vi "TimeInterpVariant_GetNewestSample.vi"(11 "TimeInterpVariant":T1) -> (1 "IsPresent":bool, 2 "TimeStamp":dbl, 3 "OutputVariant":variant)   [LabVIEW 2019, in "Trajectory_Library.lvlib"]
doc: "Get the newest sample\n\nInputs:\n - TimeInterpVariant -- Input data cluster\n\nOutputs\n - OutputVariant -- Newest Variant. \n - TimeStamp -- Time for this sample (seconds)\n - IsPresent -- Returns TRUE if the buffer contains any data"
uses:
  TypeDef/TIME_INTERPOLATABLE_VARIANT.ctl
  Trajectory_Library.lvlib
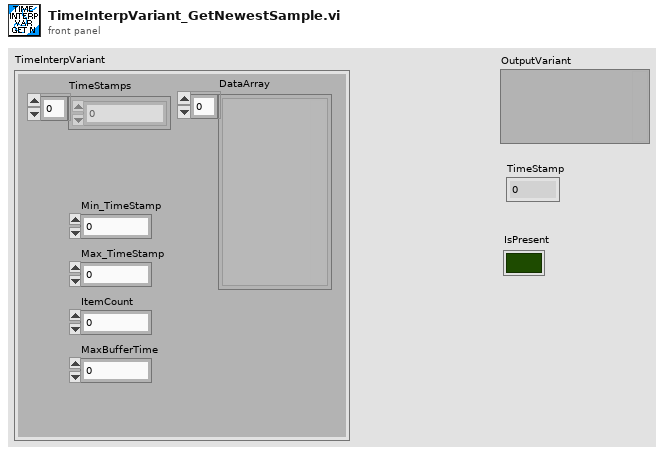
[diagram p1: front panel]
types:
  T1 = typedef "Trajectory_Library.lvlib/TIME_INTERPOLATABLE_VARIANT.ctl" = cluster{"TimeStamps":dbl[], "DataArray":variant[], "Min_TimeStamp":dbl, "Max_TimeStamp":dbl, "ItemCount":i32, "MaxBufferTime":dbl}
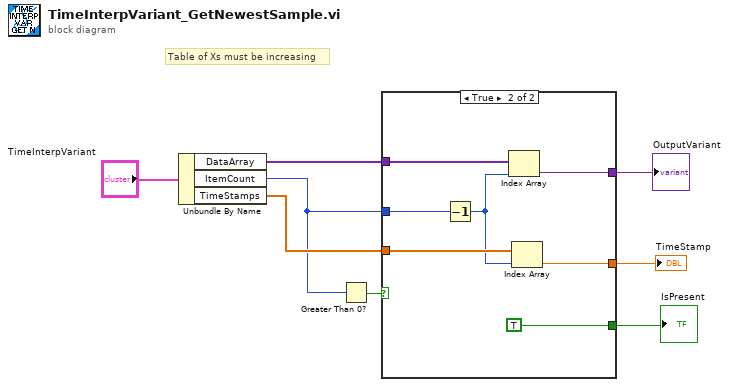
[diagram p0: block diagram]
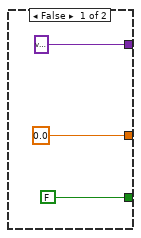
[diagram p2: hidden frame]
diagram:
  # "Table of Xs must be increasing"
  n1 = Unbundle By Name("TimeInterpVariant") -> ("DataArray"=w6:variant[], "ItemCount"=w4:i32, "TimeStamps"=w7:dbl[])
  n2 = Greater Than 0?(x=w4) -> (x > 0?=w5:bool)
  n3 = case shown="True" w5 {
    tunnel: [variant w15] -> w2
    tunnel: w4 -> [_ w13]
    tunnel: w7 -> [_ w17]
    tunnel: w6 -> [_ w18]
    tunnel: [FALSE TRUE] -> w3
    tunnel: [0.0 w16] -> w1
    frame False {
    }
    frame True {
      n4 = Decrement(x=w13) -> (x-1=w12:i32)
      n5 = Index Array(array=w18, index=w12) -> (element=w15:variant)
      n6 = Index Array(array=w17, index=w12) -> (element=w16:dbl)
    }
  }
  "OutputVariant" <- w2
  "IsPresent" <- w3
  "TimeStamp" <- w1
